vi "GPIB_comms_test.vi"(0 "Secondary address":string="1", 5 "data to write":string="READ:DEV:GRPZ:PSU:SIG:VOLT", 7 "data to write 2":string="READ:DEV:GRPZ:PSU:SIG:CURR", 9 "data to write 3":string="READ:SYS:TIME", 11 "error in":errorcluster, 13 "byte count":i32=4096, 14 "timeout ms (488.2 global)":i32=3000) -> (4 "data":string, 6 "Write Status":bool[](array[boolean]), 10 "Read Status":bool[](array[boolean]), 15 "error out":errorcluster)   [LabVIEW 2013]
panel:
  in  "Use 2nd Addr?":bool
  in  "Termination LF/CR?":bool
  in  "VISA timout (ms)":u32=2000
  in  "read-to-clear delay (ms)":u32=10
  in  "write-to-read delay (ms)":u32=10
  out "return count":u32
  in  "VISA resource name":refnum<visa-resource-name>="GPIB0::1::1::INSTR"
  in  "Use VISA?":bool
  in  "file":path=path "C:/temp/TestStrings.txt"
  out "Elapsed Seconds":i32
  in  "Primary address":string="1"
  in  "Interval between\nmessages (ms)":u32=1000
  out "Error?":bool
  in  "stop":bool
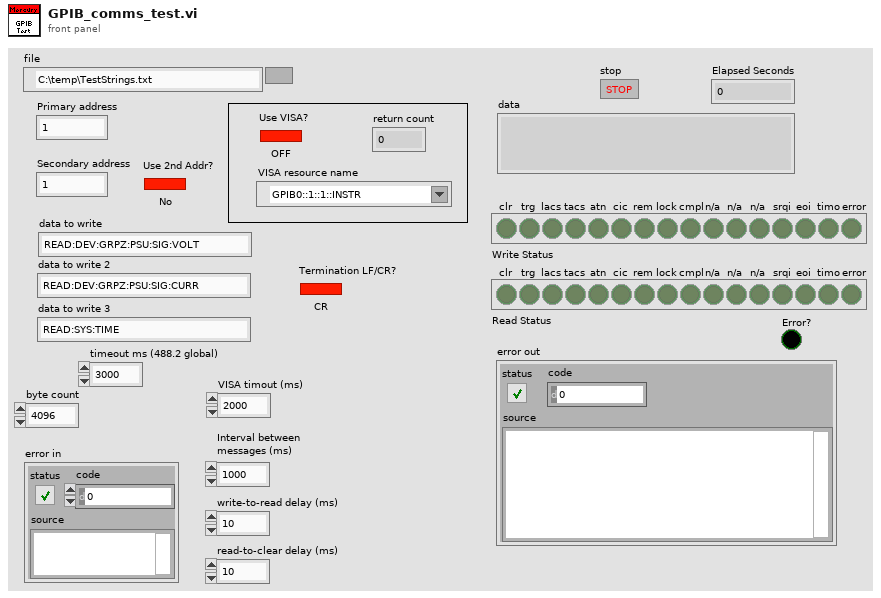
[diagram p1: front panel]
types:
  T1 = enum16{"open", "replace", "create", "open or create", "replace or create", "replace or create with confirmation"}
  T2 = typedef "LVDateTimeRec.ctl" = cluster{"fractional second":dbl, "second":i32, "minute":i32, "hour":i32, "day of month":i32, "month":i32, "year":i32, "day of week":i32, "day of year":i32, "DST":i32}
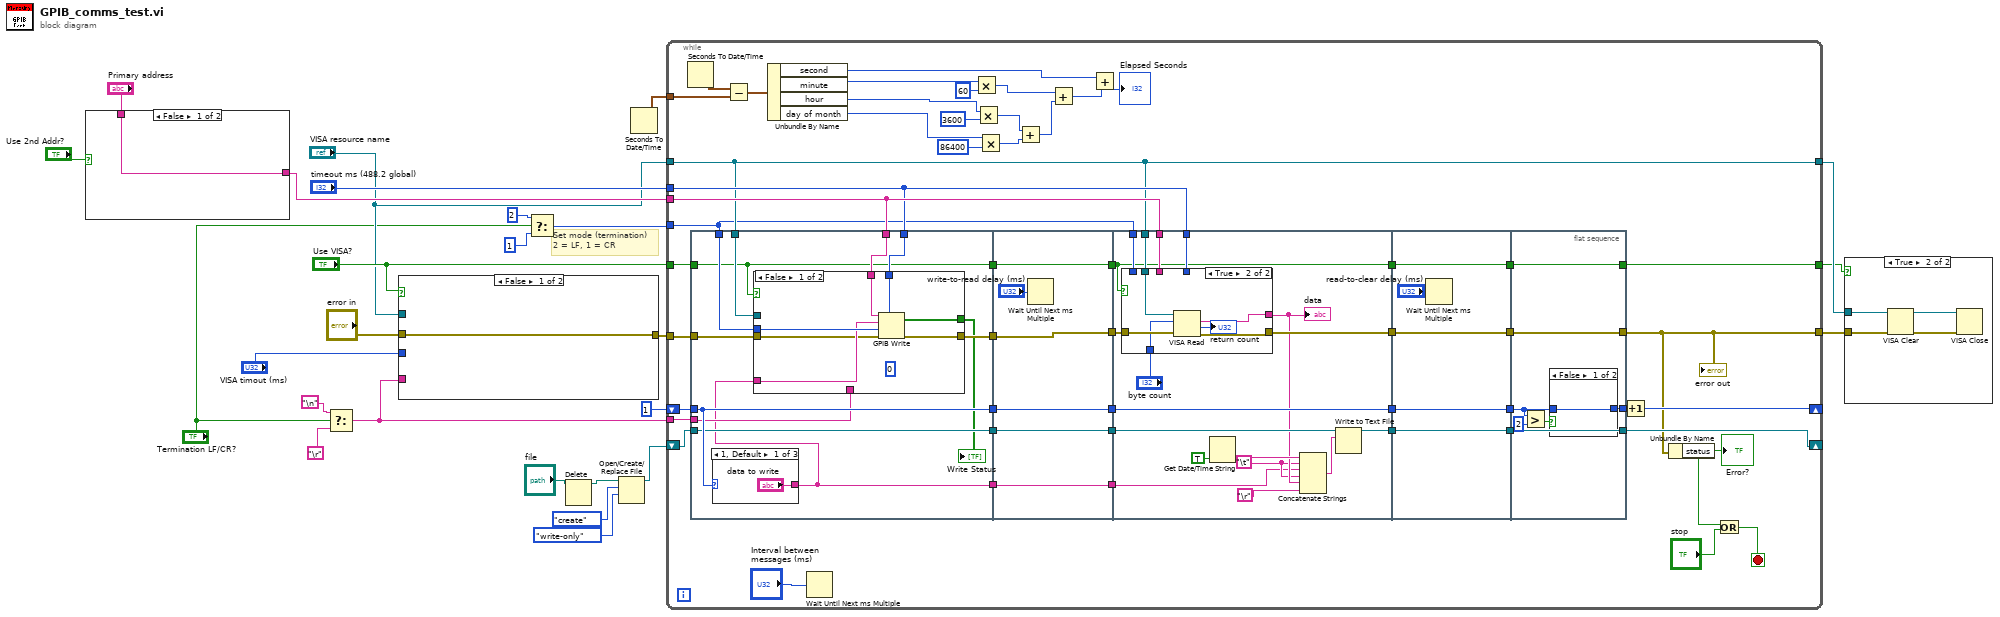
[diagram p0: block diagram]
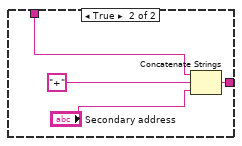
[diagram p2: hidden frame]
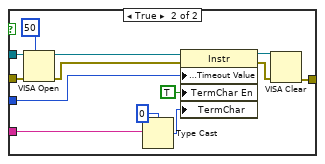
[diagram p4: hidden frame]
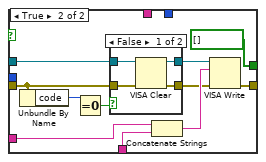
[diagram p5: hidden frame]
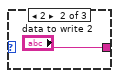
[diagram p7: hidden frame]
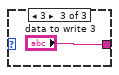
[diagram p8: hidden frame]
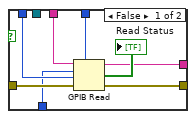
[diagram p9: hidden frame]
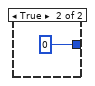
[diagram p10: hidden frame]
diagram:
  # "Set mode (termination)\n2 = LF, 1 = CR"
  n1 = case shown="False" "Use 2nd Addr?" {
    tunnel: [w27 w31] -> w25
    tunnel: "Primary address" -> [w27 w28]
    frame False {
    }
    frame True {
      n2 = Concatenate Strings(w28, "+", "Secondary address") -> (w31:string)
    }
  }
  n3 = Select(t="\n", s="Termination LF/CR?", f="\r") -> (s? t:f=w7:string)
  n4 = case shown="False" "Use VISA?" {
    tunnel: "VISA resource name" -> [_ w45]
    tunnel: "error in" -> [w32 w43]
    tunnel: [w32 w36] -> w17
    tunnel: "VISA timout (ms)" -> [_ w40]
    tunnel: w7 -> [_ w33]
    frame False {
    }
    frame True {
      n5 = VISA Open(timeout (0)=u32 50 ("VISA Open timeout (0)"), error in (no error)=w43, VISA resource name=w45) -> (VISA resource name=w44:refnum<visa-resource-name>, error out=w42:errorcluster)  [unwired: 2 in]
      n6 = Type Cast(type=u8 0 ("Message Based Settings:Termination Character"), x=w33) -> (*(type *) &x=w37:u8)
      n7 = property class="Instr"(reference=w44, error in=w42, "General Settings:Timeout Value"=w40, "TermChar En"=TRUE ("Message Based Settings:Termination Character Enable"), "TermChar"=w37) -> (reference out=w34:refnum<visa-resource-name>, error out=w35:errorcluster)
      n8 = VISA Clear(VISA resource name=w34, error in (no error)=w35) -> (error out=w36:errorcluster)  [unwired: 1 out]
    }
  }
  n9 = Select(t=i16 2 ("mode (0)"), s="Termination LF/CR?", f=i16 1 ("mode (0)")) -> (s? t:f=w3:i16)
  n10 = Delete(path (use dialog)="file") -> (deleted path=w19:path)  [unwired: 4 in, 2 out]
  n11 = Open/Create/Replace File(file path (use dialog)=w19, operation (0:open)=T1."create", access (0:read/write)=enum16{"read/write", "read-only", "write-only"}."write-only") -> (refnum out=w21:refnum<file>)  [unwired: 1 in, 4 out]
  n12 = Seconds To Date/Time() -> (date time rec=w24:T2)  [unwired: 2 in]
  n13 = while {
    shift-right: [w90] -> _
    shift-left: 1 -> [w92]
    tunnel: w17 -> [w82]
    tunnel: w25 -> [w81]
    tunnel: w24 -> [w79]
    shift-right: [w61] -> _
    shift-left: w21 -> [w64]
    tunnel: "VISA resource name" -> [w53]
    tunnel: "Use VISA?" -> [w56]
    tunnel: "timeout ms (488.2 global)" -> [w55]
    tunnel: [w54] -> w15
    tunnel: [w53] -> w14
    tunnel: [w52] -> w13
    tunnel: w7 -> [w49]
    tunnel: w3 -> [w46]
    stop <- w86 stop-if-true
    n14 = Seconds To Date/Time() -> (date time rec=w80:T2)  [unwired: 2 in]
    n15 = flat-sequence {
      tunnel: w81 -> [w109]
      tunnel: w46 -> [w108]
      tunnel: [w107] -> w97
      tunnel: w55 -> [w106]
      tunnel: [w105] -> w93
      tunnel: w92 -> [w105]
      tunnel: w82 -> [w104]
      tunnel: w64 -> [w103]
      tunnel: [w103] -> w63
      tunnel: w56 -> [w101]
      tunnel: w53 -> [w102]
      tunnel: [w101] -> w57
      tunnel: w49 -> [w99]
      tunnel: [w98] -> w47
      tunnel: [w142] -> w96
      tunnel: w97 -> [w142]
      tunnel: [w140] -> w94
      tunnel: w93 -> [w140]
      tunnel: w63 -> [w139]
      tunnel: [w139] -> w62
      tunnel: [w138] -> w58
      tunnel: w57 -> [w138]
      tunnel: [w137] -> w48
      tunnel: w47 -> [w137]
      tunnel: w81 -> [w160]
      tunnel: w46 -> [w159]
      tunnel: w96 -> [w158]
      tunnel: w55 -> [w157]
      tunnel: w94 -> [w156]
      tunnel: [w156] -> w89
      tunnel: [w155] -> w88
      tunnel: w62 -> [w153]
      tunnel: [w152] -> w59
      tunnel: w58 -> [w147]
      tunnel: w53 -> [w149]
      tunnel: [w147] -> w50
      tunnel: w48 -> [w143]
      tunnel: w89 -> [w179]
      tunnel: [w179] -> w84
      tunnel: w88 -> [w177]
      tunnel: [w177] -> w83
      tunnel: [w176] -> w60
      tunnel: w59 -> [w176]
      tunnel: [w175] -> w51
      tunnel: w50 -> [w175]
      tunnel: w84 -> [w186]
      tunnel: [w183] -> w91
      tunnel: [w182] -> w54
      tunnel: w83 -> [w182]
      tunnel: [w181] -> w61
      tunnel: w60 -> [w181]
      tunnel: [w180] -> w52
      tunnel: w51 -> [w180]
      frame #0 {
        n16 = case shown="1, Default" w105 {
          tunnel: ["data to write" "data to write 2" "data to write 3"] -> w98
          frame 1, Default {
          }
          frame 2 {
          }
          frame 3 {
          }
        }
        n17 = case shown="False" w101 {
          tunnel: w109 -> [w116 _]
          tunnel: w108 -> [w115 _]
          tunnel: [w114 w125] -> w107
          tunnel: w106 -> [w113 _]
          tunnel: w98 -> [w112 w121]
          tunnel: w104 -> [w111 w120]
          tunnel: w102 -> [_ w124]
          tunnel: [w110 bool[] [] ("status")] -> w100
          tunnel: w99 -> [_ w117]
          frame False {
            (unwired) u32 0 ("return count")
            n18 = GPIB Write(0:w116, 1:w112, 2:w115, 3:w111, 4:w113) -> (5:w110:bool[], 6:w114:errorcluster)
          }
          frame True {
            n19 = Unbundle By Name(w120) -> ("code"=w118:i32)
            n20 = Equal To 0?(x=w118) -> (x = 0?=w119:bool)
            n21 = case shown="False" w119 {
              tunnel: w124 -> [w130 w133]
              tunnel: w120 -> [w131 w132]
              tunnel: [w129 w132] -> w122
              tunnel: [w128 w133] -> w123
              frame False {
                n22 = VISA Clear(VISA resource name=w130, error in (no error)=w131) -> (VISA resource name out=w128:refnum<visa-resource-name>, error out=w129:errorcluster)
              }
              frame True {
              }
            }
            n23 = Concatenate Strings(w121, w117) -> (w127:string)
            n24 = VISA Write(VISA resource name=w123, write buffer=w127, error in (no error)=w122) -> (error out=w125:errorcluster)  [unwired: 2 out]
          }
        }
        "Write Status" <- w100
      }
      frame #1 {
        n25 = Wait Until Next ms Multiple(millisecond multiple="write-to-read delay (ms)") -> ()  [unwired: 1 out]
      }
      frame #2 {
        w144 = "\t"
        n26 = case shown="True" w147 {
          tunnel: w160 -> [w168 _]
          tunnel: w159 -> [w167 _]
          tunnel: w158 -> [w166 w174]
          tunnel: w157 -> [w165 _]
          tunnel: [w163 w173] -> w155
          tunnel: [w162 w172] -> w146
          tunnel: w149 -> [_ w171]
          tunnel: "byte count" -> [w161 w169]
          frame False {
            n27 = GPIB Read(0:w168, 1:w161, 2:w167, 3:w166, 4:w165) -> (5:w162:string, 6:→"Read Status":bool[], 7:w163:errorcluster)
          }
          frame True {
            n28 = VISA Read(VISA resource name=w171, byte count=w169, error in (no error)=w174) -> (read buffer=w172:string, return count=→"return count":u32, error out=w173:errorcluster)  [unwired: 1 out]
          }
        }
        "data" <- w146
        n29 = Get Date/Time String(want seconds? (F)=TRUE) -> (time string=w150:string)  [unwired: 2 in, 1 out]
        n30 = Concatenate Strings(w150, w144, w143, w144, w146, "\r") -> (w154:string)
        n31 = Write to Text File(file (use dialog)=w153, text=w154) -> (refnum out=w152:refnum<file>)  [unwired: 2 in, 2 out]
      }
      frame #3 {
        n32 = Wait Until Next ms Multiple(millisecond multiple="read-to-clear delay (ms)") -> ()  [unwired: 1 out]
      }
      frame #4 {
        n33 = Greater?(x=w186, y=2) -> (0:w184:bool)
        n34 = case shown="False" w184 {
          tunnel: w186 -> [w187 _]
          tunnel: [w187 0] -> w183
          frame False {
          }
          frame True {
          }
        }
      }
    }
    n35 = Subtract(x=w80, y=w79) -> (x-y=w78:T2)
    n36 = Unbundle By Name(w78) -> ("second"=w71:i32, "minute"=w77:i32, "hour"=w75:i32, "day of month"=w69:i32)
    n37 = Wait Until Next ms Multiple(millisecond multiple="Interval between\nmessages (ms)") -> ()  [unwired: 1 out]
    n38 = Multiply(x=w77, y=60) -> (x*y=w73:i32)
    n39 = Multiply(x=w75, y=3600) -> (x*y=w66:i32)
    n40 = Multiply(x=w69, y=86400) -> (x*y=w67:i32)
    n41 = Add(x=w66, y=w67) -> (x+y=w65:i32)
    n42 = Add(x=w73, y=w65) -> (x+y=w72:i32)
    n43 = Add(x=w71, y=w72) -> (x+y=→"Elapsed Seconds":i32)
    n44 = Increment(x=w91) -> (x+1=w90:i32)
    n45 = Unbundle By Name(w54) -> ("status"=w85:bool)
    "Error?" <- w85
    n46 = Or(x=w85, y="stop") -> (x .or. y?=w86:bool)
    "error out" <- w54
  }
  n47 = case shown="True" w13 {
    tunnel: w15 -> [_ w191]
    tunnel: w14 -> [_ w192]
    frame False {
    }
    frame True {
      n48 = VISA Clear(VISA resource name=w192, error in (no error)=w191) -> (VISA resource name out=w190:refnum<visa-resource-name>, error out=w189:errorcluster)
      n49 = VISA Close(VISA resource name=w190, error in (no error)=w189) -> ()  [unwired: 1 out]
    }
  }
